vi "Complete_V0.vi"() -> ()   [LabVIEW 2022 SP3]
uses:
  3bc9a862-b596-42d5-8eeb-dbbdc4778f0e.vi
  9a851694-c6f2-4fb5-8eff-591639fa9214.vi
  <vilib>/Instr/_visa.llb/VISA Configure Serial Port (Instr).vi
panel:
  out "Controller Feedback 2":string
  out "Controller Get Command Sent":string
  in  "Controller Info to Get":string(combo)
  in  "Get Controller Information":bool
  out "Adj Get Command Sent":string
  in  "Adjuster Info to Get":string(combo)
  in  "Print All Adjuster Positions":bool
  in  "Get Current Adj Information":bool
  out "Power Command Sent":string
  in  "POWER TO SYSTEM":bool
  in  "Run to end -Y":bool
  in  "Run to end +Y":bool
  in  "Run to end -X":bool
  in  "Run to end +X":bool
  in  "VISA Resource Name":refnum<visa-resource-name>
  in  "Left":bool
  in  "Down":bool
  in  "Up":bool
  in  "Right":bool
  in  "Adjustor Number":dbl format="%0#3_4p"
  in  "Emergency Stop":bool
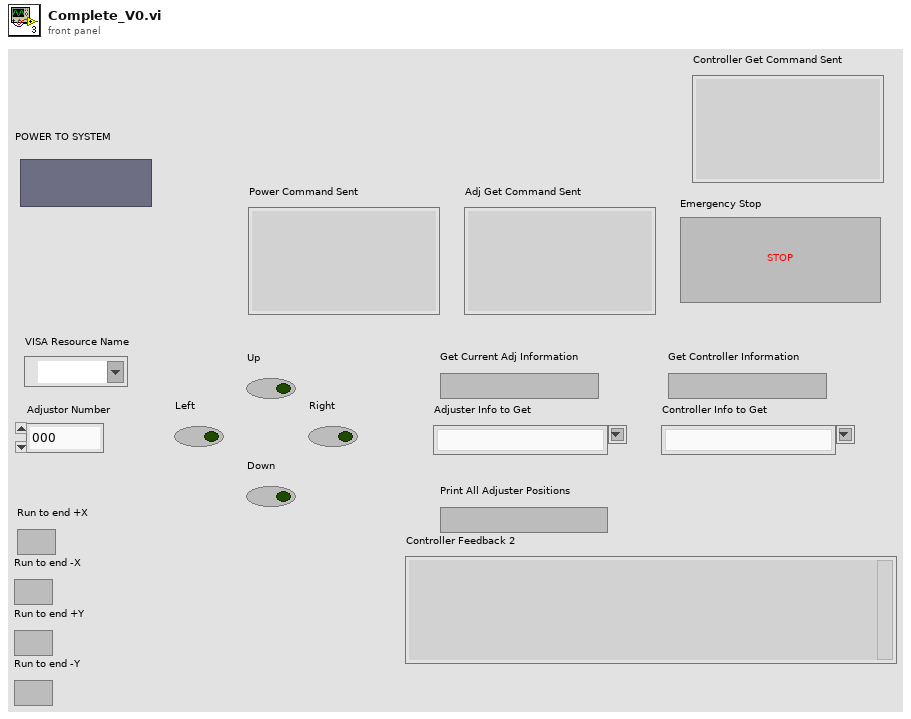
[diagram p1: front panel]
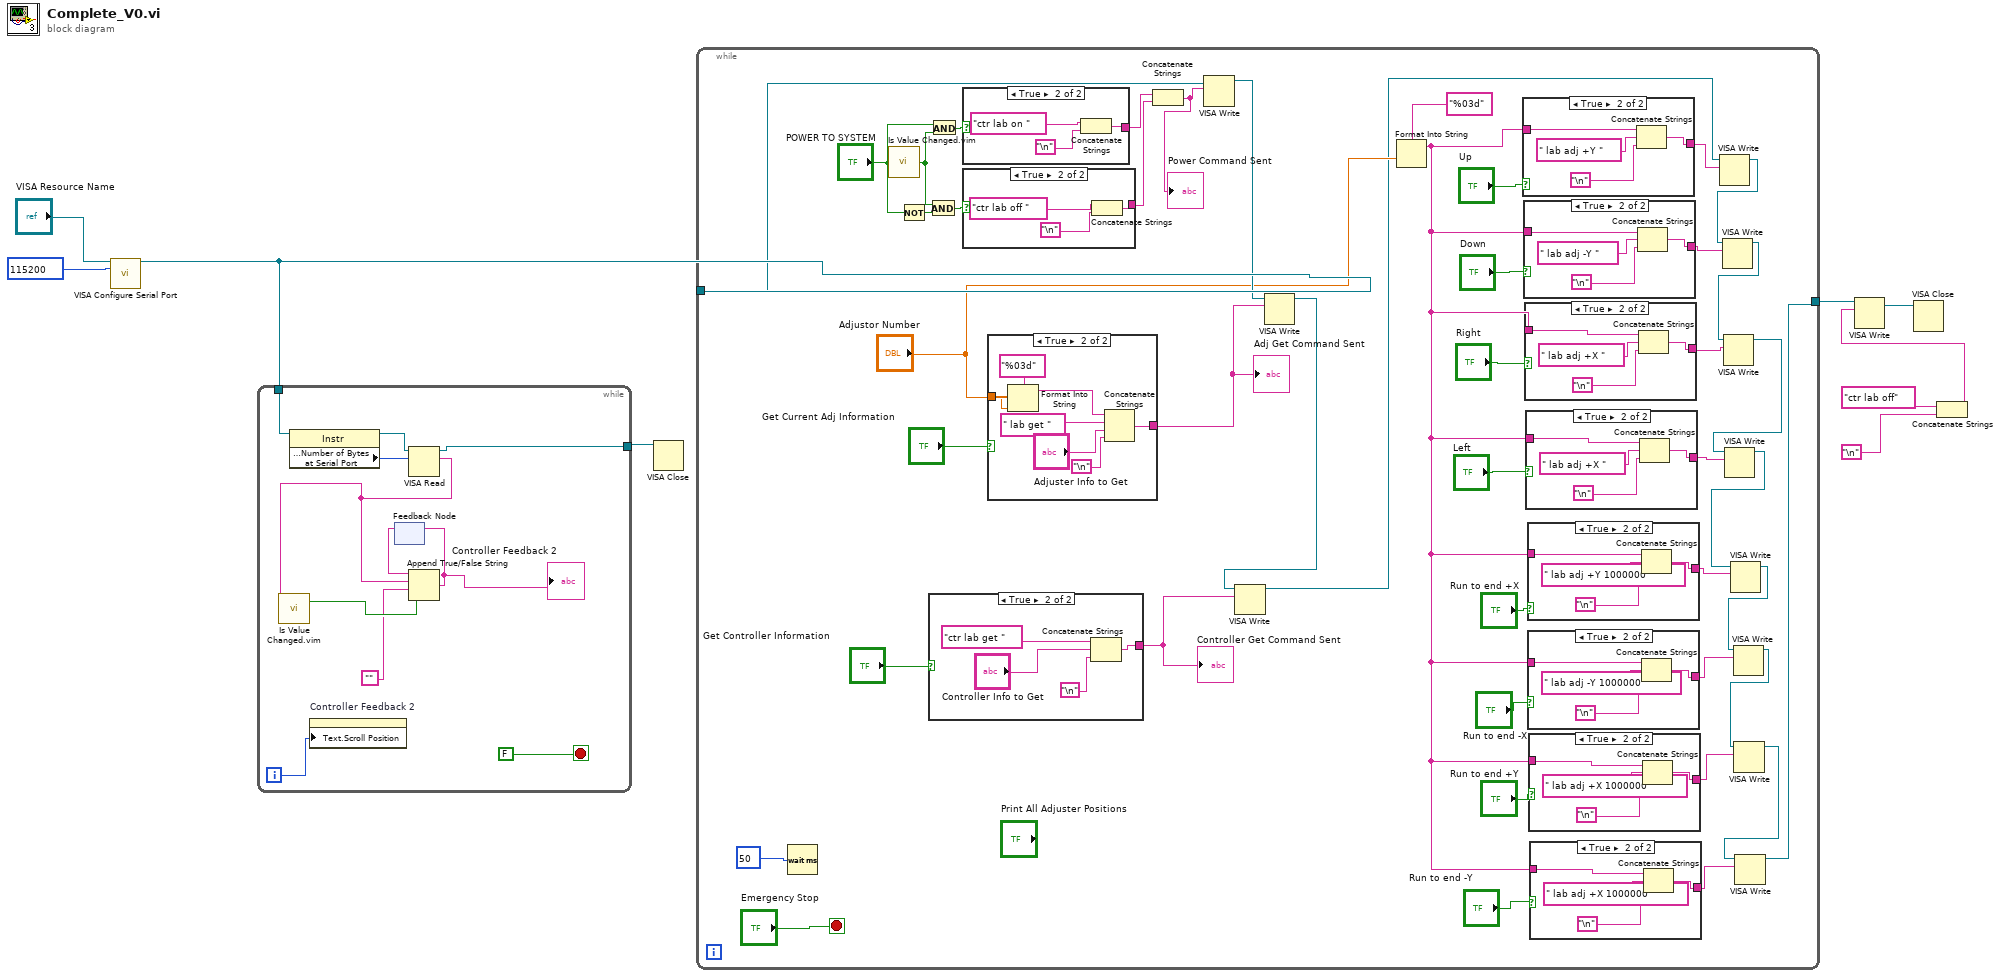
[diagram p0: block diagram]
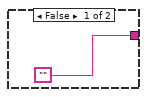
[diagram p2: hidden frame]
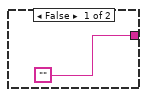
[diagram p3: hidden frame]
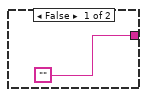
[diagram p4: hidden frame]
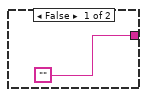
[diagram p5: hidden frame]
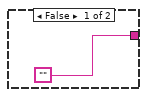
[diagram p6: hidden frame]
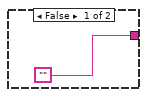
[diagram p7: hidden frame]
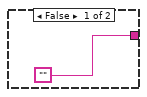
[diagram p8: hidden frame]
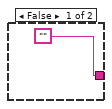
[diagram p9: hidden frame]
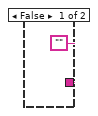
[diagram p10: hidden frame]
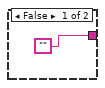
[diagram p11: hidden frame]
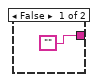
[diagram p12: hidden frame]
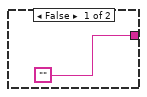
[diagram p13: hidden frame]
diagram:
  n1 = call-poly "VISA Configure Serial Port"("VISA resource name"="VISA Resource Name", "baud rate (9600)"=u32 115200) -> ("VISA resource name out"=w2:refnum<visa-resource-name>)  [unwired: 12 in, 1 out]
  n2 = while {
    tunnel: w2 -> [w13]
    tunnel: [w12] -> w1
    i -> [w10]
    stop <- FALSE stop-if-true
    n3 = property class="Instr"(reference=w13) -> (reference out=w20:refnum<visa-resource-name>, "Serial Settings:Number of Bytes at Serial Port"=w19:u32)  [unwired: 1 in, 1 out]
    n4 = property on="Controller Feedback 2" class="Str"("Text.Scroll Position"=w10) -> ()  [unwired: 2 in, 2 out]
    n5 = feedback #1() -> (w16:string)  [unwired: 1 in]
    n6 = VISA Read(VISA resource name=w20, byte count=w19) -> (VISA resource name out=w12:refnum<visa-resource-name>, read buffer=w17:string)  [unwired: 1 in, 2 out]
    n7 = call "Is Value Changed.vim"("value"=w17) -> ("changed or first call?"=w18:bool)
    n8 = Append True/False String(1:w18, 2:"", 3:w17, 4:w16) -> (0:w14:string)
    "Controller Feedback 2" <- w14
    n9 = feedback-in #1(w14) -> ()
  }
  n10 = VISA Close(VISA resource name=w1) -> ()  [unwired: 1 in, 1 out]
  n11 = while {
    tunnel: w2 -> [w63]
    tunnel: [w23] -> w8
    stop <- "Emergency Stop" stop-if-true
    n12 = Wait (ms)(milliseconds to wait=50) -> ()  [unwired: 1 out]
    n13 = call "Is Value Changed.vim"("value"="POWER TO SYSTEM") -> ("changed or first call?"=w56:bool)
    n14 = Not(x="POWER TO SYSTEM") -> (.not. x?=w61:bool)
    n15 = And(x=w56, y=w61) -> (x .and. y?=w60:bool)
    n16 = case shown="True" "Get Controller Information" {
      tunnel: ["" w102] -> w49
      frame False {
      }
      frame True {
        n17 = Concatenate Strings("ctr lab get ", "Controller Info to Get", "\n") -> (w102:string)
      }
    }
    "Controller Get Command Sent" <- w49
    n18 = And(x="POWER TO SYSTEM", y=w56) -> (x .and. y?=w62:bool)
    n19 = case shown="True" w62 {
      tunnel: ["" w120] -> w59
      frame False {
      }
      frame True {
        n20 = Concatenate Strings("ctr lab on ", "\n") -> (w120:string)
      }
    }
    n21 = case shown="True" w60 {
      tunnel: ["" w116] -> w58
      frame False {
      }
      frame True {
        n22 = Concatenate Strings("ctr lab off ", "\n") -> (w116:string)
      }
    }
    n23 = case shown="True" "Get Current Adj Information" {
      tunnel: "Adjustor Number" -> [_ w109]
      tunnel: ["" w108] -> w51
      frame False {
      }
      frame True {
        n24 = Format Into String(format string="%03d", w109) -> (resulting string=w107:string)  [unwired: 2 in, 1 out]
        n25 = Concatenate Strings(w107, " lab get ", "Adjuster Info to Get", "\n") -> (w108:string)
      }
    }
    "Adj Get Command Sent" <- w51
    n26 = Concatenate Strings(w59, w58) -> (w55:string)
    "Power Command Sent" <- w55
    n27 = VISA Write(VISA resource name=w63, write buffer=w55) -> (VISA resource name out=w53:refnum<visa-resource-name>)  [unwired: 1 in, 2 out]
    n28 = VISA Write(VISA resource name=w53, write buffer=w51) -> (VISA resource name out=w48:refnum<visa-resource-name>)  [unwired: 1 in, 2 out]
    n29 = VISA Write(VISA resource name=w48, write buffer=w49) -> (VISA resource name out=w47:refnum<visa-resource-name>)  [unwired: 1 in, 2 out]
    n30 = Format Into String(format string="%03d", "Adjustor Number") -> (resulting string=w32:string)  [unwired: 2 in, 1 out]
    n31 = case shown="True" "Up" {
      tunnel: ["" w123] -> w46
      tunnel: w32 -> [_ w126]
      frame False {
      }
      frame True {
        n32 = Concatenate Strings(w126, " lab adj +Y ", "\n") -> (w123:string)
      }
    }
    n33 = case shown="True" "Down" {
      tunnel: ["" w97] -> w44
      tunnel: w32 -> [_ w100]
      frame False {
      }
      frame True {
        n34 = Concatenate Strings(w100, " lab adj -Y ", "\n") -> (w97:string)
      }
    }
    n35 = case shown="True" "Right" {
      tunnel: ["" w92] -> w42
      tunnel: w32 -> [_ w95]
      frame False {
      }
      frame True {
        n36 = Concatenate Strings(w95, " lab adj +X ", "\n") -> (w92:string)
      }
    }
    n37 = case shown="True" "Left" {
      tunnel: ["" w87] -> w38
      tunnel: w32 -> [_ w90]
      frame False {
      }
      frame True {
        n38 = Concatenate Strings(w90, " lab adj +X ", "\n") -> (w87:string)
      }
    }
    n39 = case shown="True" "Run to end +X" {
      tunnel: ["" w82] -> w31
      tunnel: w32 -> [_ w85]
      frame False {
      }
      frame True {
        n40 = Concatenate Strings(w85, " lab adj +Y 1000000 ", "\n") -> (w82:string)
      }
    }
    n41 = case shown="True" "Run to end -X" {
      tunnel: ["" w77] -> w28
      tunnel: w32 -> [_ w80]
      frame False {
      }
      frame True {
        n42 = Concatenate Strings(w80, " lab adj -Y 1000000 ", "\n") -> (w77:string)
      }
    }
    n43 = case shown="True" "Run to end +Y" {
      tunnel: ["" w72] -> w26
      tunnel: w32 -> [_ w75]
      frame False {
      }
      frame True {
        n44 = Concatenate Strings(w75, " lab adj +X 1000000 ", "\n") -> (w72:string)
      }
    }
    n45 = case shown="True" "Run to end -Y" {
      tunnel: ["" w67] -> w24
      tunnel: w32 -> [_ w70]
      frame False {
      }
      frame True {
        n46 = Concatenate Strings(w70, " lab adj +X 1000000 ", "\n") -> (w67:string)
      }
    }
    n47 = VISA Write(VISA resource name=w47, write buffer=w46) -> (VISA resource name out=w43:refnum<visa-resource-name>)  [unwired: 1 in, 2 out]
    n48 = VISA Write(VISA resource name=w43, write buffer=w44) -> (VISA resource name out=w40:refnum<visa-resource-name>)  [unwired: 1 in, 2 out]
    n49 = VISA Write(VISA resource name=w40, write buffer=w42) -> (VISA resource name out=w37:refnum<visa-resource-name>)  [unwired: 1 in, 2 out]
    n50 = VISA Write(VISA resource name=w37, write buffer=w38) -> (VISA resource name out=w30:refnum<visa-resource-name>)  [unwired: 1 in, 2 out]
    n51 = VISA Write(VISA resource name=w30, write buffer=w31) -> (VISA resource name out=w29:refnum<visa-resource-name>)  [unwired: 1 in, 2 out]
    n52 = VISA Write(VISA resource name=w29, write buffer=w28) -> (VISA resource name out=w27:refnum<visa-resource-name>)  [unwired: 1 in, 2 out]
    n53 = VISA Write(VISA resource name=w27, write buffer=w26) -> (VISA resource name out=w25:refnum<visa-resource-name>)  [unwired: 1 in, 2 out]
    n54 = VISA Write(VISA resource name=w25, write buffer=w24) -> (VISA resource name out=w23:refnum<visa-resource-name>)  [unwired: 1 in, 2 out]
  }
  n55 = Concatenate Strings("ctr lab off", "\n") -> (w4:string)
  n56 = VISA Write(VISA resource name=w8, write buffer=w4) -> (VISA resource name out=w7:refnum<visa-resource-name>)  [unwired: 1 in, 2 out]
  n57 = VISA Close(VISA resource name=w7) -> ()  [unwired: 1 in, 1 out]
